vi "IMAQ DLL - Non Zero Indices.vi"(0 "IMAQ Ref":T1, 11 "Error In":errorcluster) -> (4 "IMAQ Ref (Dup)":T1, 8 "Row Column Indices":i32[][](array[numeric]), 13 "Non Zero Px Total":u16, 15 "Error Out":errorcluster)   [LabVIEW 2020]
uses:
  <vilib>/vision/Image Controls.llb/IMAQ Image.ctl
  LabView IMAQ Images DLL Files/x64/Release/LabView IMAQ Images.dll
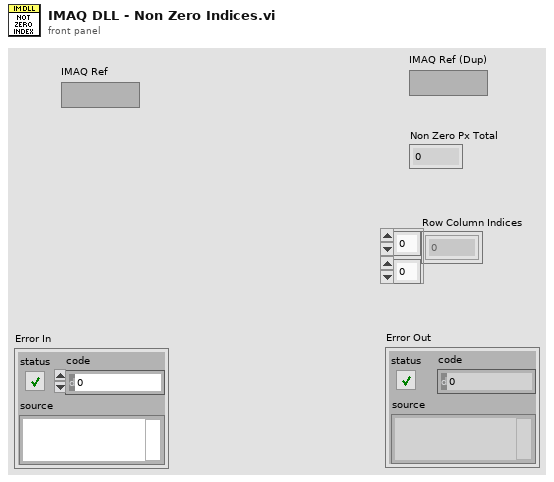
[diagram p1: front panel]
types:
  T1 = typedef "IMAQ Image.ctl" = refnum<image>
  T2 = enum32{"Map Pixel Pointer", "Unmap Pixel Pointer", "Get Pixels Infos"}
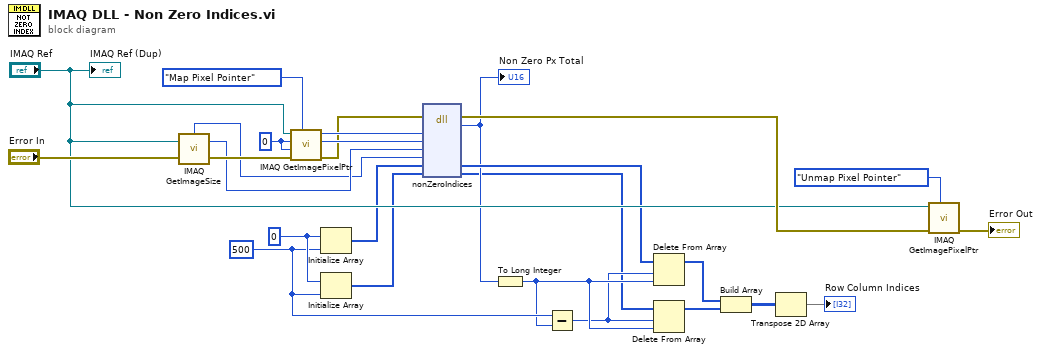
[diagram p0: block diagram]
diagram:
  w9 = 500 ("dimension size")
  w12 = 0 ("element")
  w24 = 0 ("X Coordinate")
  n1 = call "IMAQ GetImageSize"("Image"="IMAQ Ref", "error in (no error)"="Error In") -> ("Y Resolution"=w22:i32, "X Resolution"=w21:i32, "error out"=w26:errorcluster)  [unwired: 2 in]
  n2 = call "IMAQ GetImagePixelPtr"("Function"=T2."Map Pixel Pointer", "error in (no error)"=w26, "Y Coordinate"=w24, "X Coordinate"=w24, "Image"="IMAQ Ref") -> ("error out"=w20:errorcluster, "LineWidth(Pixels)"=w23:i32, "Pixel Pointer out"=w25:u64)  [unwired: 1 in, 3 out]
  n3 = Initialize Array(w12, w9) -> (w13:i32[])
  n4 = Initialize Array(w12, w9) -> (w11:i32[])
  n5 = dll-call lib="C:/Users/George Sirinakis/Documents/Microscope-Control/Tools/LabView IMAQ Images/LabView IMAQ Images DLL Files/x64/Release/LabView IMAQ Images.dll" fn="nonZeroIndices"(error in=w20, "imPointer"=w25, "LV_Line_Width"=w23, "LV_Rows"=w22, "LV_Cols"=w21, "Row Indices"=w13, "Col Indices"=w11) -> (error out=w17:errorcluster, "numNotZero"=w8:u16, "Row Indices"=w10:i32[], "Col Indices"=w1:i32[])  [unwired: 6 in, 1 out]
  "Non Zero Px Total" <- w8
  n6 = To Long Integer(number=w8) -> (32bit integer=w7:i32)
  n7 = Subtract(x=w9, y=w7) -> (x-y=w6:i32)
  n8 = Delete From Array(array=w10, length=w6, index=w7) -> (array with subset deleted=w5:i32[])  [unwired: 1 out]
  n9 = Delete From Array(array=w1, length=w6, index=w7) -> (array with subset deleted=w4:i32[])  [unwired: 1 out]
  n10 = Build Array(w5, w4) -> (w3:i32[][])
  n11 = Transpose 2D Array(2D array=w3) -> (transposed array=→"Row Column Indices":i32[][])
  n12 = call "IMAQ GetImagePixelPtr"("Function"=T2."Unmap Pixel Pointer", "error in (no error)"=w17, "Image"="IMAQ Ref") -> ("error out"=→"Error Out":errorcluster)  [unwired: 3 in, 5 out]
  "IMAQ Ref (Dup)" <- "IMAQ Ref"
